vi "WildDrive_v5.vi"(8 "Super Turn":bool, 10 "Turn Joystick":dbl, 11 "Speed Joystick":dbl) -> (0 "Right Side Power":dbl, 3 "Left Side Power":dbl)   [LabVIEW 2018]
uses:
  <vilib>/Analysis/1siggen.llb/Ramp Pattern by Samples.vi
  <vilib>/Analysis/NI_AALBase.lvlib
panel:
  out "Mixing Function":cluster{"Y":dbl[], "X":dbl[]}(graph)={"Y"=[0.0, 0.010101010101010102, 0.020202020202020204, 0.030303030303030304, 0.04040404040404041, 0.05050505050505051, 0.06060606060606061, 0.07070707070707072, 0.08080808080808081, 0.09090909090909091, 0.10101010101010102, 0.11111111111111112, 0.12121212121212122, 0.13131313131313133, 0.14141414141414144, 0.15151515151515152, 0.16161616161616163, 0.17171717171717174, 0.18181818181818182, 0.19191919191919193, 0.20202020202020204, 0.21212121212121213, 0.22222222222222224, 0.23232323232323235, 0.24242424242424243, 0.25252525252525254, 0.26262626262626265, 0.27272727272727276, 0.2828282828282829, 0.29292929292929293, 0.30303030303030304, 0.31313131313131315, 0.32323232323232326, 0.33333333333333337, 0.3434343434343435, 0.3535353535353536, 0.36363636363636365, 0.37373737373737376, 0.38383838383838387, 0.393939393939394, 0.4040404040404041, 0.4141414141414142, 0.42424242424242425, 0.43434343434343436, 0.4444444444444445, 0.4545454545454546, 0.4646464646464647, 0.4747474747474748, 0.48484848484848486, 0.494949494949495, 0.5050505050505051, 0.5151515151515152, 0.5252525252525253, 0.5353535353535354, 0.5454545454545455, 0.5555555555555556, 0.5656565656565657, 0.5757575757575758, 0.5858585858585859, 0.595959595959596, 0.6060606060606061, 0.6161616161616162, 0.6262626262626263, 0.6363636363636365, 0.6464646464646465, 0.6565656565656566, 0.6666666666666667, 0.6767676767676768, 0.686868686868687, 0.696969696969697, 0.7070707070707072, 0.7171717171717172, 0.7272727272727273, 0.7373737373737375, 0.7474747474747475, 0.7575757575757577, 0.7676767676767677, 0.7777777777777778, 0.787878787878788, 0.797979797979798, 0.8080808080808082, 0.8181818181818182, 0.8282828282828284, 0.8383838383838385, 0.8484848484848485, 0.8585858585858587, 0.8686868686868687, 0.8787878787878789, 0.888888888888889, 0.8989898989898991, 0.9090909090909092, 0.9191919191919192, 0.9292929292929294, 0.9393939393939394, 0.9494949494949496, 0.9595959595959597, 0.9696969696969697, 0.9797979797979799, 0.98989898989899, 1.0], "X"=[1.0, 0.739700373388279, 0.5488006593124598, 0.4083670427152411, 0.30474675984494354, 0.2280634338225159, 0.17114998516436622, 0.12878932884527872, 0.09717230561019187, 0.07350944999341955, 0.05575205753661255, 0.04239115827521615, 0.0323121959854341, 0.024689662756899957, 0.018910479166168403, 0.014518117194448454, 0.011171735048430028, 0.008616207734047168, 0.00666008827578714, 0.005159357462919659, 0.0040054101696625, 0.0031161507293951296, 0.0024293759535134745, 0.0018978457763698243, 0.0014856020661604733, 0.0011652128973970383, 0.0009157047092917002, 0.0007210070053945374, 0.0005687798590093595, 0.00044952800045262425, 0.00035592994620023085, 0.00028232885622580476, 0.00022434529622522844, 0.00017858209017001413, 0.00014239889161561293, 0.00011373964986286524, 9.100029141270006e-05, 7.292704004463544e-05, 5.853812709502422e-05, 4.706339427721292e-05, 3.789761070744471e-05, 3.0564322083219484e-05, 2.468780385551084e-05, 1.9971261874998804e-05, 1.6179858305474368e-05, 1.3127471227072999e-05, 1.0666348540777324e-05, 8.679009512968307e-06, 7.071894863511227e-06, 5.770379497061955e-06, 4.714848969430282e-06, 3.857607756366577e-06, 3.160439049156962e-06, 2.5926757139178352e-06, 2.1296729433931007e-06, 1.7515970812202518e-06, 1.4424636999795213e-06, 1.1893724850068803e-06, 9.818977518046873e-07, 8.116022255915986e-07, 6.71648591462865e-07, 5.564887105401966e-07, 4.6161462199150505e-07, 3.833587688511337e-07, 3.18733495650665e-07, 2.6530192213582984e-07, 2.2107391972073306e-07, 1.844221992542213e-07, 1.5401453306014844e-07, 1.2875893805057942e-07, 1.0775928460418692e-07, 9.02793028178225e-08, 7.571336112837868e-08, 6.356271374653796e-08, 5.341616983618422e-08, 4.49343423108951e-08, 3.783679808043171e-08, 3.1891562929491325e-08, 2.6906539570420593e-08, 2.2722482031298726e-08, 1.9207237588962195e-08, 1.6251022246560417e-08, 1.3762539924527316e-08, 1.1665791184537986e-08, 9.897446115616289e-09, 8.404679320520214e-09, 7.1433838212844356e-09, 6.076696014397879e-09, 5.173776237527475e-09, 4.408799614224464e-09, 3.760120065458747e-09, 3.2095770751417075e-09, 2.7419202595359222e-09, 2.3443312503774242e-09, 2.006026046670479e-09, 1.7179239724894285e-09, 1.4723718208143653e-09, 1.2629137661884245e-09, 1.084099272741887e-09, 9.313225746154785e-10]}
  in  "Mixing Coefficient":dbl(slide)=30.0 min=1.0 max=100.0 scale=1.0..100.0
  in  "Debug Mode":bool
  in  "Debug Speed":dbl(slide) min=0.0 max=1.0 scale=0.0..1.0
  in  "Square Speed":bool=TRUE
  in  "Feed Forward Coeff":dbl(slide)=0.05 min=0.0 max=0.2 scale=0.0..0.2
  in  "Max Pivot Turn (super)":dbl(slide)=1.0 min=0.0 max=1.0 scale=0.0..1.0
  in  "Max Pivot Turn (normal)":dbl(slide)=0.5 min=0.0 max=1.0 scale=0.0..1.0
  in  "Tune Arc Turn":dbl(slide)=1.2 min=0.9 max=2.0 scale=0.9..2.0
  in  "Speed Joystick Deadband":dbl(slide)=0.05 min=0.0 max=1.0 scale=0.0..1.0
  in  "Turn Behavior":bool=TRUE
  out "Left Side Power":cluster{"Y":dbl[], "X":dbl[]}(graph)={"Y"=[0.0, 0.010101010101010102, 0.020202020202020204, 0.030303030303030304, 0.04040404040404041, 0.05050505050505051, 0.06060606060606061, 0.07070707070707072, 0.08080808080808081, 0.09090909090909091, 0.10101010101010102, 0.11111111111111112, 0.12121212121212122, 0.13131313131313133, 0.14141414141414144, 0.15151515151515152, 0.16161616161616163, 0.17171717171717174, 0.18181818181818182, 0.19191919191919193, 0.20202020202020204, 0.21212121212121213, 0.22222222222222224, 0.23232323232323235, 0.24242424242424243, 0.25252525252525254, 0.26262626262626265, 0.27272727272727276, 0.2828282828282829, 0.29292929292929293, 0.30303030303030304, 0.31313131313131315, 0.32323232323232326, 0.33333333333333337, 0.3434343434343435, 0.3535353535353536, 0.36363636363636365, 0.37373737373737376, 0.38383838383838387, 0.393939393939394, 0.4040404040404041, 0.4141414141414142, 0.42424242424242425, 0.43434343434343436, 0.4444444444444445, 0.4545454545454546, 0.4646464646464647, 0.4747474747474748, 0.48484848484848486, 0.494949494949495, 0.5050505050505051, 0.5151515151515152, 0.5252525252525253, 0.5353535353535354, 0.5454545454545455, 0.5555555555555556, 0.5656565656565657, 0.5757575757575758, 0.5858585858585859, 0.595959595959596, 0.6060606060606061, 0.6161616161616162, 0.6262626262626263, 0.6363636363636365, 0.6464646464646465, 0.6565656565656566, 0.6666666666666667, 0.6767676767676768, 0.686868686868687, 0.696969696969697, 0.7070707070707072, 0.7171717171717172, 0.7272727272727273, 0.7373737373737375, 0.7474747474747475, 0.7575757575757577, 0.7676767676767677, 0.7777777777777778, 0.787878787878788, 0.797979797979798, 0.8080808080808082, 0.8181818181818182, 0.8282828282828284, 0.8383838383838385, 0.8484848484848485, 0.8585858585858587, 0.8686868686868687, 0.8787878787878789, 0.888888888888889, 0.8989898989898991, 0.9090909090909092, 0.9191919191919192, 0.9292929292929294, 0.9393939393939394, 0.9494949494949496, 0.9595959595959597, 0.9696969696969697, 0.9797979797979799, 0.98989898989899, 1.0], "X"=[0.0]}
  out "Right Side Power":cluster{"Y":dbl[], "X":dbl[]}(graph)={"Y"=[0.0, 0.010101010101010102, 0.020202020202020204, 0.030303030303030304, 0.04040404040404041, 0.05050505050505051, 0.06060606060606061, 0.07070707070707072, 0.08080808080808081, 0.09090909090909091, 0.10101010101010102, 0.11111111111111112, 0.12121212121212122, 0.13131313131313133, 0.14141414141414144, 0.15151515151515152, 0.16161616161616163, 0.17171717171717174, 0.18181818181818182, 0.19191919191919193, 0.20202020202020204, 0.21212121212121213, 0.22222222222222224, 0.23232323232323235, 0.24242424242424243, 0.25252525252525254, 0.26262626262626265, 0.27272727272727276, 0.2828282828282829, 0.29292929292929293, 0.30303030303030304, 0.31313131313131315, 0.32323232323232326, 0.33333333333333337, 0.3434343434343435, 0.3535353535353536, 0.36363636363636365, 0.37373737373737376, 0.38383838383838387, 0.393939393939394, 0.4040404040404041, 0.4141414141414142, 0.42424242424242425, 0.43434343434343436, 0.4444444444444445, 0.4545454545454546, 0.4646464646464647, 0.4747474747474748, 0.48484848484848486, 0.494949494949495, 0.5050505050505051, 0.5151515151515152, 0.5252525252525253, 0.5353535353535354, 0.5454545454545455, 0.5555555555555556, 0.5656565656565657, 0.5757575757575758, 0.5858585858585859, 0.595959595959596, 0.6060606060606061, 0.6161616161616162, 0.6262626262626263, 0.6363636363636365, 0.6464646464646465, 0.6565656565656566, 0.6666666666666667, 0.6767676767676768, 0.686868686868687, 0.696969696969697, 0.7070707070707072, 0.7171717171717172, 0.7272727272727273, 0.7373737373737375, 0.7474747474747475, 0.7575757575757577, 0.7676767676767677, 0.7777777777777778, 0.787878787878788, 0.797979797979798, 0.8080808080808082, 0.8181818181818182, 0.8282828282828284, 0.8383838383838385, 0.8484848484848485, 0.8585858585858587, 0.8686868686868687, 0.8787878787878789, 0.888888888888889, 0.8989898989898991, 0.9090909090909092, 0.9191919191919192, 0.9292929292929294, 0.9393939393939394, 0.9494949494949496, 0.9595959595959597, 0.9696969696969697, 0.9797979797979799, 0.98989898989899, 1.0], "X"=[0.0]}
  in  "Turn Joystick Deadband":dbl(slide)=0.05 min=0.0 max=1.0 scale=0.0..1.0
  out "Speed Joystick Mapping":cluster{"Y":dbl[], "X":dbl[]}(graph)={"Y"=[0.0, 0.010101010101010102, 0.020202020202020204, 0.030303030303030304, 0.04040404040404041, 0.05050505050505051, 0.06060606060606061, 0.07070707070707072, 0.08080808080808081, 0.09090909090909091, 0.10101010101010102, 0.11111111111111112, 0.12121212121212122, 0.13131313131313133, 0.14141414141414144, 0.15151515151515152, 0.16161616161616163, 0.17171717171717174, 0.18181818181818182, 0.19191919191919193, 0.20202020202020204, 0.21212121212121213, 0.22222222222222224, 0.23232323232323235, 0.24242424242424243, 0.25252525252525254, 0.26262626262626265, 0.27272727272727276, 0.2828282828282829, 0.29292929292929293, 0.30303030303030304, 0.31313131313131315, 0.32323232323232326, 0.33333333333333337, 0.3434343434343435, 0.3535353535353536, 0.36363636363636365, 0.37373737373737376, 0.38383838383838387, 0.393939393939394, 0.4040404040404041, 0.4141414141414142, 0.42424242424242425, 0.43434343434343436, 0.4444444444444445, 0.4545454545454546, 0.4646464646464647, 0.4747474747474748, 0.48484848484848486, 0.494949494949495, 0.5050505050505051, 0.5151515151515152, 0.5252525252525253, 0.5353535353535354, 0.5454545454545455, 0.5555555555555556, 0.5656565656565657, 0.5757575757575758, 0.5858585858585859, 0.595959595959596, 0.6060606060606061, 0.6161616161616162, 0.6262626262626263, 0.6363636363636365, 0.6464646464646465, 0.6565656565656566, 0.6666666666666667, 0.6767676767676768, 0.686868686868687, 0.696969696969697, 0.7070707070707072, 0.7171717171717172, 0.7272727272727273, 0.7373737373737375, 0.7474747474747475, 0.7575757575757577, 0.7676767676767677, 0.7777777777777778, 0.787878787878788, 0.797979797979798, 0.8080808080808082, 0.8181818181818182, 0.8282828282828284, 0.8383838383838385, 0.8484848484848485, 0.8585858585858587, 0.8686868686868687, 0.8787878787878789, 0.888888888888889, 0.8989898989898991, 0.9090909090909092, 0.9191919191919192, 0.9292929292929294, 0.9393939393939394, 0.9494949494949496, 0.9595959595959597, 0.9696969696969697, 0.9797979797979799, 0.98989898989899, 1.0], "X"=[0.0]}
  out "Turn Joystick Mapping":cluster{"Y":dbl[], "X":dbl[]}(graph)={"Y"=[0.0, 0.010101010101010102, 0.020202020202020204, 0.030303030303030304, 0.04040404040404041, 0.05050505050505051, 0.06060606060606061, 0.07070707070707072, 0.08080808080808081, 0.09090909090909091, 0.10101010101010102, 0.11111111111111112, 0.12121212121212122, 0.13131313131313133, 0.14141414141414144, 0.15151515151515152, 0.16161616161616163, 0.17171717171717174, 0.18181818181818182, 0.19191919191919193, 0.20202020202020204, 0.21212121212121213, 0.22222222222222224, 0.23232323232323235, 0.24242424242424243, 0.25252525252525254, 0.26262626262626265, 0.27272727272727276, 0.2828282828282829, 0.29292929292929293, 0.30303030303030304, 0.31313131313131315, 0.32323232323232326, 0.33333333333333337, 0.3434343434343435, 0.3535353535353536, 0.36363636363636365, 0.37373737373737376, 0.38383838383838387, 0.393939393939394, 0.4040404040404041, 0.4141414141414142, 0.42424242424242425, 0.43434343434343436, 0.4444444444444445, 0.4545454545454546, 0.4646464646464647, 0.4747474747474748, 0.48484848484848486, 0.494949494949495, 0.5050505050505051, 0.5151515151515152, 0.5252525252525253, 0.5353535353535354, 0.5454545454545455, 0.5555555555555556, 0.5656565656565657, 0.5757575757575758, 0.5858585858585859, 0.595959595959596, 0.6060606060606061, 0.6161616161616162, 0.6262626262626263, 0.6363636363636365, 0.6464646464646465, 0.6565656565656566, 0.6666666666666667, 0.6767676767676768, 0.686868686868687, 0.696969696969697, 0.7070707070707072, 0.7171717171717172, 0.7272727272727273, 0.7373737373737375, 0.7474747474747475, 0.7575757575757577, 0.7676767676767677, 0.7777777777777778, 0.787878787878788, 0.797979797979798, 0.8080808080808082, 0.8181818181818182, 0.8282828282828284, 0.8383838383838385, 0.8484848484848485, 0.8585858585858587, 0.8686868686868687, 0.8787878787878789, 0.888888888888889, 0.8989898989898991, 0.9090909090909092, 0.9191919191919192, 0.9292929292929294, 0.9393939393939394, 0.9494949494949496, 0.9595959595959597, 0.9696969696969697, 0.9797979797979799, 0.98989898989899, 1.0], "X"=[-0.0]}
  # "Driver Inputs"
  # "Tuning Parameters"
  # "Debug"
  # "Drive Outputs"
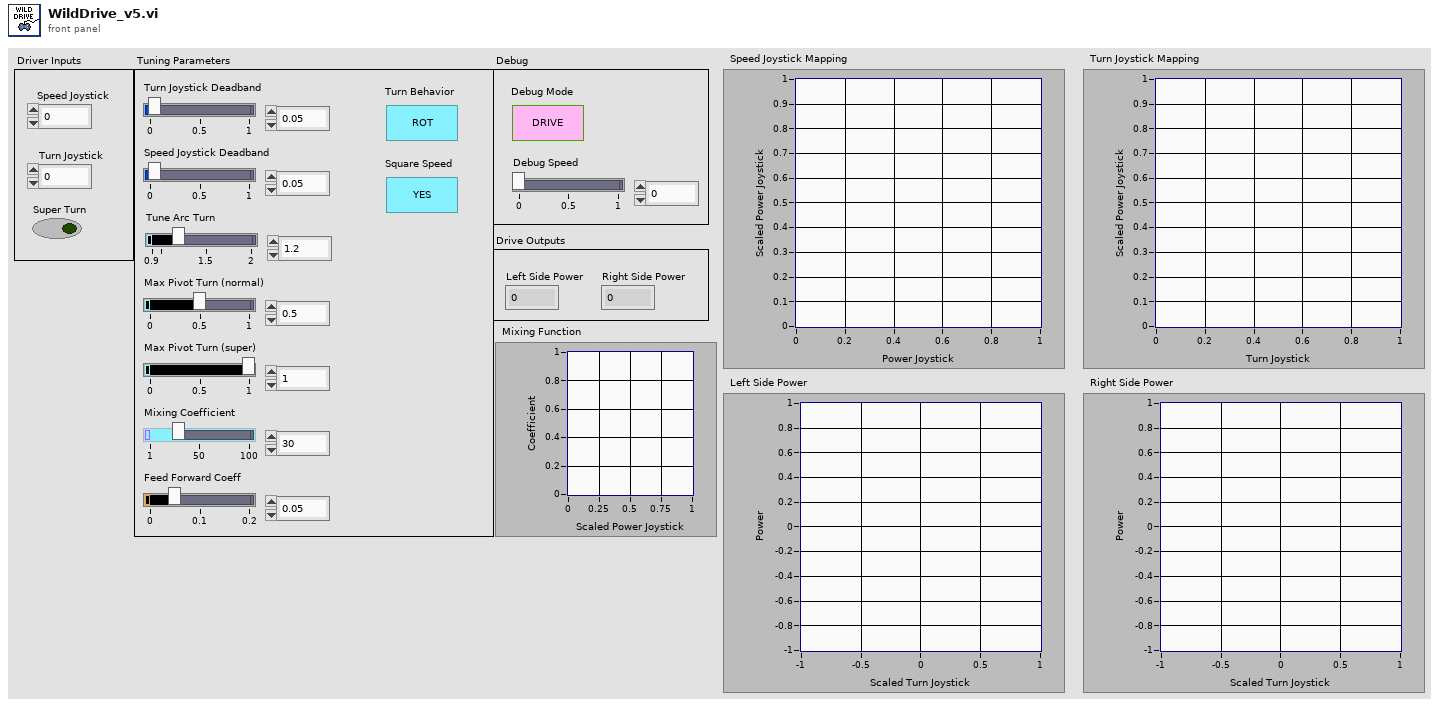
[diagram p1: front panel]
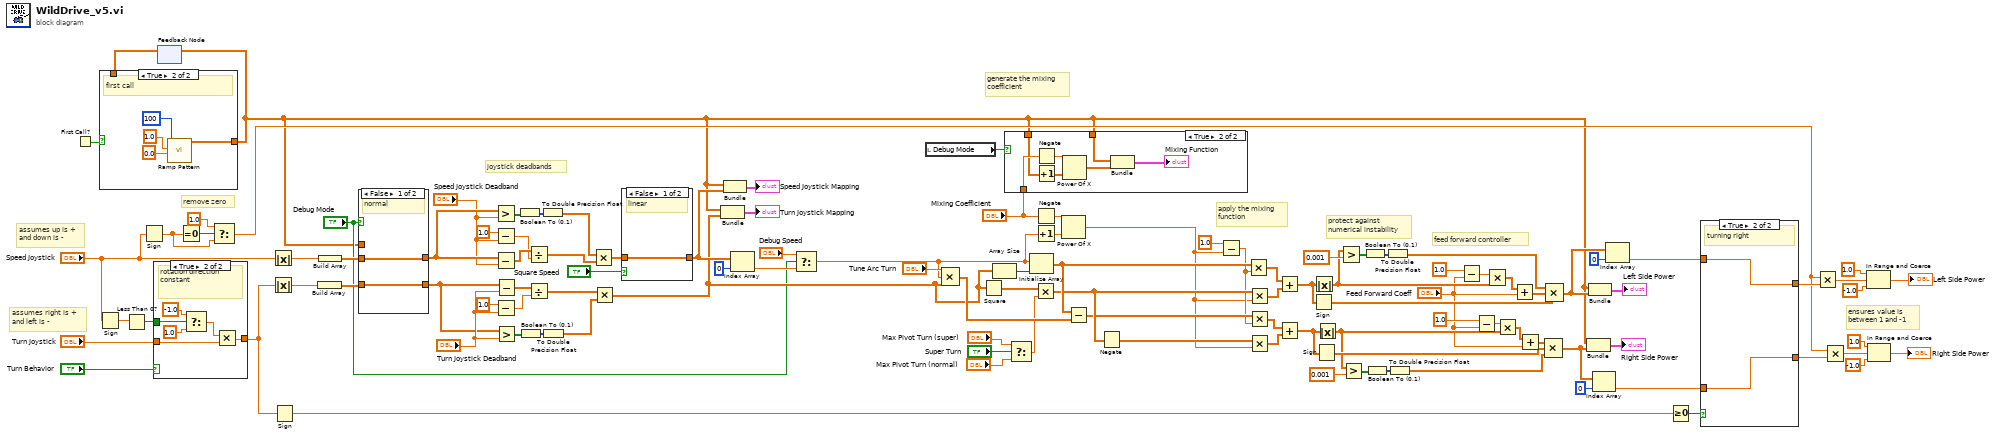
[diagram p0: block diagram]
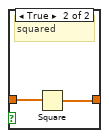
[diagram p7: hidden frame]
diagram:
  # "assumes right is +\nand left is -"
  # "assumes up is +\nand down is -"
  # "apply the mixing\nfunction"
  # "generate the mixing\ncoefficient"
  # "remove zero"
  # "protect against\nnumerical instability"
  # "ensures value is \nbetween 1 and -1"
  # "feed forward controller"
  # "joystick deadbands"
  n1 = First Call?() -> (First Call?: T/F=w32:bool)
  n2 = Sign(1:"Speed Joystick") -> (0:w42:dbl)
  n3 = Less Than 0?(x=w42) -> (x < 0?=w43:bool)
  n4 = Sign(1:"Speed Joystick") -> (0:w35:dbl)
  n5 = case shown="True" "Turn Behavior" {
    tunnel: w43 -> [_ w118]
    tunnel: [w113 w115] -> w38
    tunnel: "Turn Joystick" -> [w113 w114]
    frame False {
      # "like a car"
    }
    frame True {
      # "rotation direction constant"
      n6 = Select(t=-1.0, s=w118, f=1.0) -> (s? t:f=w119:dbl)
      n7 = Multiply(x=w119, y=w114) -> (x*y=w115:dbl)
    }
  }
  n8 = feedback #1() -> (w31:dbl[])  [unwired: 1 in]
  n9 = case shown="True" w32 {
    tunnel: [w120 w121] -> w2
    tunnel: w31 -> [w120 _]
    frame False {
      # "subsequent calls"
    }
    frame True {
      # "first call"
      n10 = call-poly <vilib>:"Ramp Pattern.vi"("start"=0.0, "end"=1.0, "samples"=100) -> ("Ramp Pattern"=w121:dbl[])  [unwired: 7 in, 1 out]
    }
  }
  n11 = feedback-in #1(w2) -> ()
  n12 = Equal To 0?(x=w35) -> (x = 0?=w37:bool)
  n13 = Select(t=1.0, s=w37, f=w35) -> (s? t:f=w34:dbl)
  n14 = Absolute Value(x="Speed Joystick") -> (abs(x)=w109:dbl)
  n15 = Absolute Value(x=w38) -> (abs(x)=w112:dbl)
  n16 = Sign(1:w38) -> (0:w46:dbl)
  n17 = Build Array(w112) -> (w110:dbl[])
  n18 = Build Array(w109) -> (w111:dbl[])
  n19 = case shown="False" "Debug Mode" {
    tunnel: w2 -> [_ w127]
    tunnel: [w126 w127] -> w100
    tunnel: [w125 w127] -> w91
    tunnel: w111 -> [w126 _]
    tunnel: w110 -> [w125 _]
    frame False {
      # "normal"
    }
    frame True {
      # "debug"
    }
  }
  n20 = Greater?(x=w100, y="Speed Joystick Deadband") -> (0:w106:bool[])
  n21 = Subtract(x=1.0, y="Speed Joystick Deadband") -> (x-y=w97:dbl)
  n22 = Subtract(x=w100, y="Speed Joystick Deadband") -> (x-y=w99:dbl[])
  n23 = Subtract(x=1.0, y="Turn Joystick Deadband") -> (x-y=w93:dbl)
  n24 = Subtract(x=w91, y="Turn Joystick Deadband") -> (x-y=w95:dbl[])
  n25 = Greater?(x=w91, y="Turn Joystick Deadband") -> (0:w104:bool[])
  n26 = Boolean To (0,1)(Boolean=w106) -> (0, 1=w105:i16[])
  n27 = Boolean To (0,1)(Boolean=w104) -> (0, 1=w103:i16[])
  n28 = Divide(x=w99, y=w97) -> (x/y=w96:dbl[])
  n29 = Divide(x=w95, y=w93) -> (x/y=w90:dbl[])
  n30 = To Double Precision Float(number=w105) -> (double precision float=w102:dbl[])
  n31 = To Double Precision Float(number=w103) -> (double precision float=w89:dbl[])
  n32 = Multiply(x=w102, y=w96) -> (x*y=w101:dbl[])
  n33 = Multiply(x=w90, y=w89) -> (x*y=w22:dbl[])
  n34 = case shown="False" "Square Speed" {
    tunnel: w101 -> [w128 w130]
    tunnel: [w128 w129] -> w82
    frame False {
      # "linear"
    }
    frame True {
      # "squared"
      n35 = Square(x=w130) -> (x^2=w129:dbl[])
    }
  }
  n36 = Bundle("Ramp Pattern"=w2, w22) -> (→"Turn Joystick Mapping":cluster{"Ramp Pattern":dbl[], dbl[]})  [unwired: 1 in]
  n37 = Bundle("Ramp Pattern"=w2, w82) -> (→"Speed Joystick Mapping":cluster{"Ramp Pattern":dbl[], dbl[]})  [unwired: 1 in]
  n38 = Index Array(array=w82, index=0) -> (element=w84:dbl)
  n39 = Select(t="Debug Speed", s="Debug Mode", f=w84) -> (s? t:f=w7:dbl)
  n40 = local read "Debug Mode"() -> (w1:bool)
  n41 = Compound Arithmetic op=MULTIPLY("Tune Arc Turn", w7, w22) -> (w85:dbl[])
  n42 = Square(x=w22) -> (x^2=w33:dbl[])
  n43 = Array Size(array=w22) -> (size(s)=w88:i32)
  n44 = case shown="True" w1 {
    tunnel: "Mixing Coefficient" -> [_ w135]
    tunnel: w2 -> [_ w133]
    tunnel: w2 -> [_ w131]
    frame False {
    }
    frame True {
      n45 = Negate(x=w135) -> (-x=w137:dbl)
      n46 = Increment(x=w133) -> (x+1=w136:dbl[])
      n47 = Power Of X(1:w136, 2:w137) -> (0:w132:dbl[])
      n48 = Bundle("Ramp Pattern"=w131, w132) -> (→"Mixing Function":cluster{"Ramp Pattern":dbl[], dbl[]})  [unwired: 1 in]
    }
  }
  n49 = Select(t="Max Pivot Turn (super)", s="Super Turn", f="Max Pivot Turn (normal)") -> (s? t:f=w30:dbl)
  n50 = Initialize Array(w7, w88) -> (w19:dbl[])
  n51 = Multiply(x=w33, y=w30) -> (x*y=w18:dbl[])
  n52 = Negate(x="Mixing Coefficient") -> (-x=w6:dbl)
  n53 = Increment(x=w7) -> (x+1=w5:dbl)
  n54 = Power Of X(1:w5, 2:w6) -> (0:w4:dbl)
  n55 = Subtract(x=w19, y=w85) -> (x-y=w12:dbl[])
  n56 = Negate(x=w18) -> (-x=w11:dbl[])
  n57 = Subtract(x=1.0, y=w4) -> (x-y=w8:dbl)
  n58 = Multiply(x=w19, y=w8) -> (x*y=w17:dbl[])
  n59 = Multiply(x=w18, y=w4) -> (x*y=w16:dbl[])
  n60 = Multiply(x=w12, y=w8) -> (x*y=w14:dbl[])
  n61 = Multiply(x=w11, y=w4) -> (x*y=w13:dbl[])
  n62 = Add(x=w17, y=w16) -> (x+y=w15:dbl[])
  n63 = Add(x=w14, y=w13) -> (x+y=w10:dbl[])
  n64 = Sign(1:w15) -> (0:w78:dbl[])
  n65 = Absolute Value(x=w15) -> (abs(x)=w44:dbl[])
  n66 = Sign(1:w10) -> (0:w73:dbl[])
  n67 = Absolute Value(x=w10) -> (abs(x)=w45:dbl[])
  n68 = Greater?(x=w44, y=0.001) -> (0:w68:bool[])
  n69 = Greater?(x=w45, y=0.001) -> (0:w72:bool[])
  n70 = Boolean To (0,1)(Boolean=w68) -> (0, 1=w67:i16[])
  n71 = Boolean To (0,1)(Boolean=w72) -> (0, 1=w71:i16[])
  n72 = To Double Precision Float(number=w67) -> (double precision float=w65:dbl[])
  n73 = To Double Precision Float(number=w71) -> (double precision float=w69:dbl[])
  n74 = Subtract(x=1.0, y="Feed Forward Coeff") -> (x-y=w80:dbl)
  n75 = Subtract(x=1.0, y="Feed Forward Coeff") -> (x-y=w76:dbl)
  n76 = Multiply(x=w80, y=w44) -> (x*y=w79:dbl[])
  n77 = Multiply(x=w76, y=w45) -> (x*y=w75:dbl[])
  n78 = Add(x=w79, y="Feed Forward Coeff") -> (x+y=w64:dbl[])
  n79 = Add(x=w75, y="Feed Forward Coeff") -> (x+y=w74:dbl[])
  n80 = Compound Arithmetic op=MULTIPLY(w74, w73, w69) -> (w62:dbl[])
  n81 = Compound Arithmetic op=MULTIPLY(w65, w64, w78) -> (w60:dbl[])
  n82 = Bundle("Ramp Pattern"=w2, w62) -> (→"Right Side Power":cluster{"Ramp Pattern":dbl[], dbl[]})  [unwired: 1 in]
  n83 = Bundle("Ramp Pattern"=w2, w60) -> (→"Left Side Power":cluster{"Ramp Pattern":dbl[], dbl[]})  [unwired: 1 in]
  n84 = Index Array(array=w62, index=0) -> (element=w49:dbl)
  n85 = Index Array(array=w60, index=0) -> (element=w51:dbl)
  n86 = Greater Or Equal To 0?(x=w46) -> (x >= 0?=w47:bool)
  n87 = case shown="True" w47 {
    tunnel: w51 -> [w139 w141]
    tunnel: [w138 w141] -> w50
    tunnel: w49 -> [w138 w140]
    tunnel: [w139 w140] -> w48
    frame False {
      # "turning left"
    }
    frame True {
      # "turning right"
    }
  }
  n88 = Multiply(x=w34, y=w50) -> (x*y=w52:dbl)
  n89 = Multiply(x=w34, y=w48) -> (x*y=w53:dbl)
  n90 = In Range and Coerce(upper limit=1.0, x=w52, lower limit=-1.0) -> (coerced(x)=→"Left Side Power":dbl)  [unwired: 1 out]
  n91 = In Range and Coerce(upper limit=1.0, x=w53, lower limit=-1.0) -> (coerced(x)=→"Right Side Power":dbl)  [unwired: 1 out]
